vi "Process of Out-of-range Devices.vi"(0 "Range Check Results":T1(array[cluster]), 1 "State File Refnum":refnum<file>, 2 "Recipients":string[](array[string]), 5 "Devices":refnum<class "ACNET Devices.lvclass">, 7 "Monitoring Listbox":refnum<vi>, 9 "Summary Listbox":refnum<vi>, 11 "error in (no error)":errorcluster, 12 "Out-of-Range Alert Sound File":path=path "C:/Users/plane/Dropbox/Research/MTA/DAQ VIs/MTA Shift Toolbox/alertklaxon_clean.wav", 13 "Back-in-Range Alert Sound File":path=path "C:/Users/plane/Dropbox/Research/MTA/DAQ VIs/MTA Shift Toolbox/tng-data-allsystems.wav") -> (4 "State Changed":bool, 15 "error out":errorcluster)   [LabVIEW 2013, in "ACNET Monitor.lvlib"]
uses:
  ACNET Monitor.lvlib
  ACNET Devices.lvclass
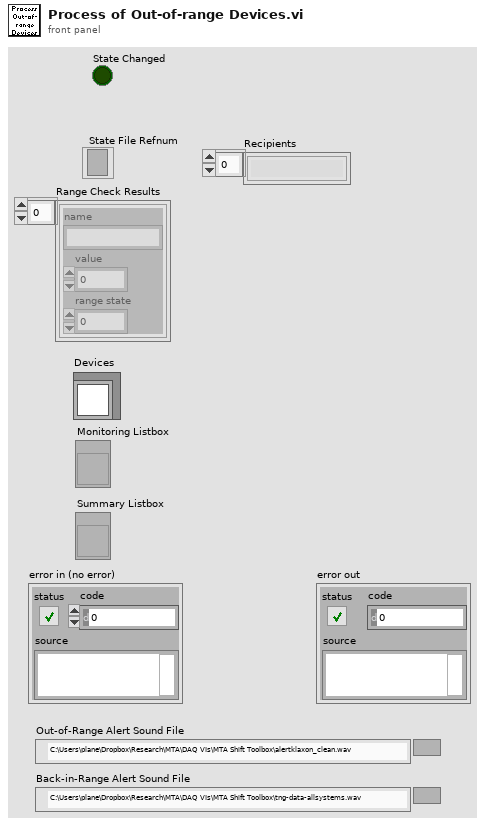
[diagram p1: front panel]
types:
  T1 = cluster{"name":string, "value":dbl, "range state":i8}[]
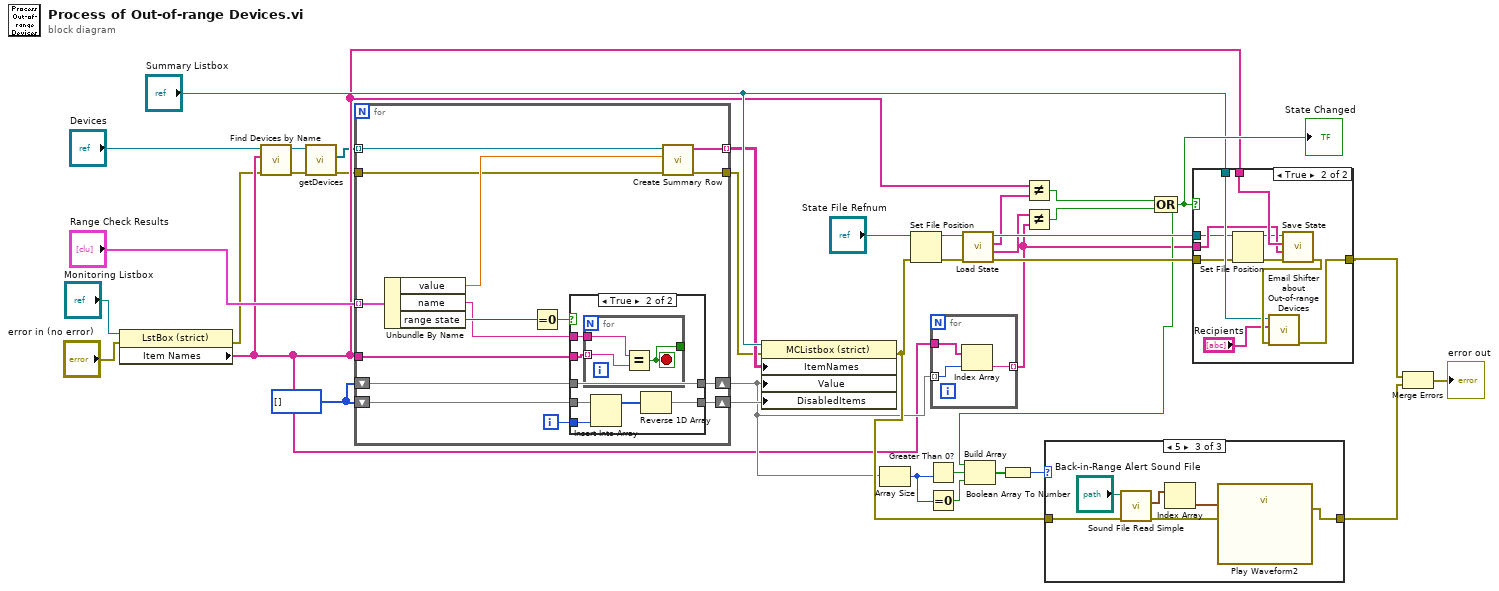
[diagram p0: block diagram]
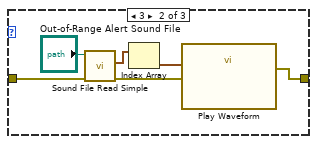
[diagram p4: hidden frame]
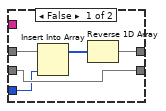
[diagram p5: hidden frame]
diagram:
  w36 = i32[] [] ("Disabled Items")
  n1 = property on="Property Node" class="LstBox (strict)"(reference="Monitoring Listbox", error in="error in (no error)") -> (error out=w5:errorcluster, "Item Names"=w6:string[])  [unwired: 1 out]
  n2 = call "Find Devices by Name.vi"("error in"=w5, "Device Names"=w6, "ACNET Devices in"="Devices") -> ("error out"=w4:errorcluster, "ACNET Devices out"=w2:refnum<class "ACNET Devices.lvclass">)  [unwired: 7 in]
  n3 = call-dynamic "getDevices.vi"("error in (no error)"=w4, "ACNET Devices in"=w2) -> ("error out"=w3:errorcluster, "Devices"=w1:refnum<class "ACNET Device.lvclass">[])  [unwired: 7 in, 1 out]
  n4 = for {
    tunnel: "Range Check Results" -> [w51] mode=indexing
    tunnel: w6 -> [w48]
    shift-right: [w45] -> w32
    shift-left: w36 -> [w47]
    shift-right: [w43] -> w11
    shift-left: w36 -> [w44]
    tunnel: w1 -> [w41] mode=indexing
    tunnel: [w40] -> w9 mode=indexing
    tunnel: w3 -> [w38]
    tunnel: [w37] -> w8
    i -> [w46]
    n5 = Unbundle By Name(w51) -> ("value"=w39:dbl, "name"=w42:string, "range state"=w50:i8)
    n6 = Equal To 0?(x=w50) -> (x = 0?=w49:bool)
    n7 = case shown="True" w49 {
      tunnel: w48 -> [_ w63]
      tunnel: w42 -> [_ w62]
      tunnel: w47 -> [w56 w61]
      tunnel: w46 -> [w53 w60]
      tunnel: [w56 w58] -> w45
      tunnel: w44 -> [w54 w57]
      tunnel: [w52 w57] -> w43
      frame False {
        n8 = Insert Into Array(array=w54, new element=w53) -> (w55:i32[])  [unwired: 1 in]
        n9 = Reverse 1D Array(array=w55) -> (reversed array=w52:i32[])
      }
      frame True {
        n10 = for {
          tunnel: w63 -> [w66] mode=indexing
          tunnel: w62 -> [w65]
          tunnel: [w64] -> _
          stop <- w64 stop-if-true
          n11 = Equal?(x=w65, y=w66) -> (x = y?=w64:bool)
        }
        n12 = Insert Into Array(array=w61, new element=w60) -> (w59:i32[])  [unwired: 1 in]
        n13 = Reverse 1D Array(array=w59) -> (reversed array=w58:i32[])
      }
    }
    n14 = call "Create Summary Row.vi"("error in (no error)"=w38, "value"=w39, "ACNET Device.lvclass"=w41) -> ("error out"=w37:errorcluster, "Summary Row"=w40:string[])  [unwired: 7 in]
  }
  n15 = property on="Property Node" class="MCListbox (strict)"(reference="Summary Listbox", error in=w8, "ItemNames"=w9, "Value"=w11, "DisabledItems"=w32) -> (error out=w27:errorcluster)  [unwired: 1 out]
  n16 = Array Size(array=w11) -> (size(s)=w23:i32)
  n17 = Set File Position(refnum="State File Refnum", error in=w27) -> (refnum out=w14:refnum<file>, error out=w15:errorcluster)  [unwired: 2 in]
  n18 = Greater Than 0?(x=w23) -> (x > 0?=w25:bool)
  n19 = Equal To 0?(x=w23) -> (x = 0?=w24:bool)
  n20 = for {
    tunnel: w11 -> [w69] mode=indexing
    tunnel: w6 -> [w68]
    tunnel: [w67] -> w18 mode=indexing
    n21 = Index Array(array=w68, index=w69) -> (element=w67:string)
  }
  n22 = call "Load State.vi"("error in"=w15, "State File Refnum"=w14) -> ("error out"=w29:errorcluster, "Out-of-range List"=w16:string[], "Monitoring List"=w17:string[], "refnum out"=w28:refnum<file>)  [unwired: 6 in]
  n23 = Not Equal?(x=w6, y=w17) -> (x != y?=w31:bool)
  n24 = Not Equal?(x=w16, y=w18) -> (x != y?=w30:bool)
  n25 = Compound Arithmetic op=OR(w31, w30) -> (w26:bool)
  "State Changed" <- w26
  n26 = Build Array(w26, w25, w24) -> (w22:bool[])
  n27 = Boolean Array To Number(Boolean array=w22) -> (number=w21:u32)
  n28 = case shown="5" w21 {
    tunnel: w27 -> [w70 w72 w78]
    tunnel: [w70 w71 w77] -> w19
    frame 0, Default {
    }
    frame 3 {
      n29 = call <vilib>:"Sound File Read Simple.vi"("error in (no error)"=w72, "path"="Out-of-Range Alert Sound File") -> ("error out"=w74:errorcluster, "data"=w76:waveform(dbl)[])  [unwired: 6 in, 2 out]
      n30 = Index Array(array=w76) -> (element=w75:waveform(dbl))  [unwired: 1 in]
      n31 = call "Play Waveform"("Data"=w75, "error in"=w74) -> ("error out"=w71:errorcluster)  [unwired: 17 in]
    }
    frame 5 {
      n32 = call <vilib>:"Sound File Read Simple.vi"("error in (no error)"=w78, "path"="Back-in-Range Alert Sound File") -> ("error out"=w80:errorcluster, "data"=w82:waveform(dbl)[])  [unwired: 6 in, 2 out]
      n33 = Index Array(array=w82) -> (element=w81:waveform(dbl))  [unwired: 1 in]
      n34 = call "Play Waveform2"("Data"=w81, "error in"=w80) -> ("error out"=w77:errorcluster)  [unwired: 17 in]
    }
  }
  n35 = case shown="True" w26 {
    tunnel: w29 -> [w83 w86]
    tunnel: [w83 w92] -> w12
    tunnel: w28 -> [_ w88]
    tunnel: "Summary Listbox" -> [_ w91]
    tunnel: w6 -> [_ w90]
    tunnel: w18 -> [_ w89]
    frame False {
    }
    frame True {
      n36 = Set File Position(refnum=w88, error in=w86) -> (refnum out=w87:refnum<file>, error out=w85:errorcluster)  [unwired: 2 in]
      n37 = call "Save State.vi"("error in"=w85, "Out-of-range List"=w89, "Monitoring List"=w90, "State File Refnum in"=w87) -> ("error out"=w93:errorcluster)  [unwired: 6 in, 1 out]
      n38 = call "Email Shifter about Out-of-range Devices.vi"("error in"=w93, "Recipients"="Recipients", "Summary Listbox"=w91) -> ("error out"=w92:errorcluster)  [unwired: 8 in]
    }
  }
  n39 = Merge Errors(w12, w19) -> (→"error out":errorcluster)
